vi "Robot Main.vi"() -> ()   [LabVIEW 2011]
doc: "This VI imlements the framework and scheduler for your robotics program. It should not be necessary to modify the framework. You are expected to add your code to the VIs called from Robot Main, the ones located in the Team Code within the project."
uses:
  <vilib>/Rock Robotics/WPI/Camera/WPI_CameraImageSize.ctl
  Robot Global Data.vi
panel:
  in  "Image Size":T1=enum."320x240"
  in  "Enable Vision":bool=TRUE
  in  "Finish":bool
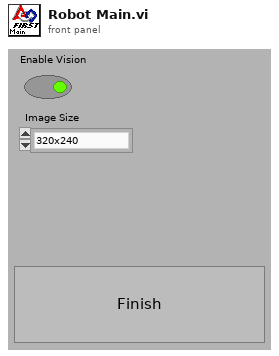
[diagram p1: front panel]
types:
  T1 = typedef "WPI_CameraImageSize.ctl" = enum16{"640x480", "320x240", "160x120"}
  T2 = typedef "WPI_DriverStationMatch Info.ctl" = cluster{"Autonomous Elapsed Seconds":dbl, "TeleOp Elapsed Seconds":dbl, "Disabled Elapsed Seconds":dbl, "Visited Autonomous":bool, "Visited TeleOp":bool, "Visited Disabled":bool, "Autonomous Settings":cluster{"Autonomous Style":enum16{"Iterative", "Independent"}, "VI Refnum":refnum<vi>}}
  T3 = typedef "WPI_DriverStationDerivedRobotMode.ctl" = enum16{"Init", "Execute", "Stop"}
  T4 = typedef "WPI_DriverStationRobotMode.ctl" = enum16{"Autonomous Disabled", "Autonomous Enabled", "Teleop Disabled", "Teleop Enabled", "Timeout", "Finish"}
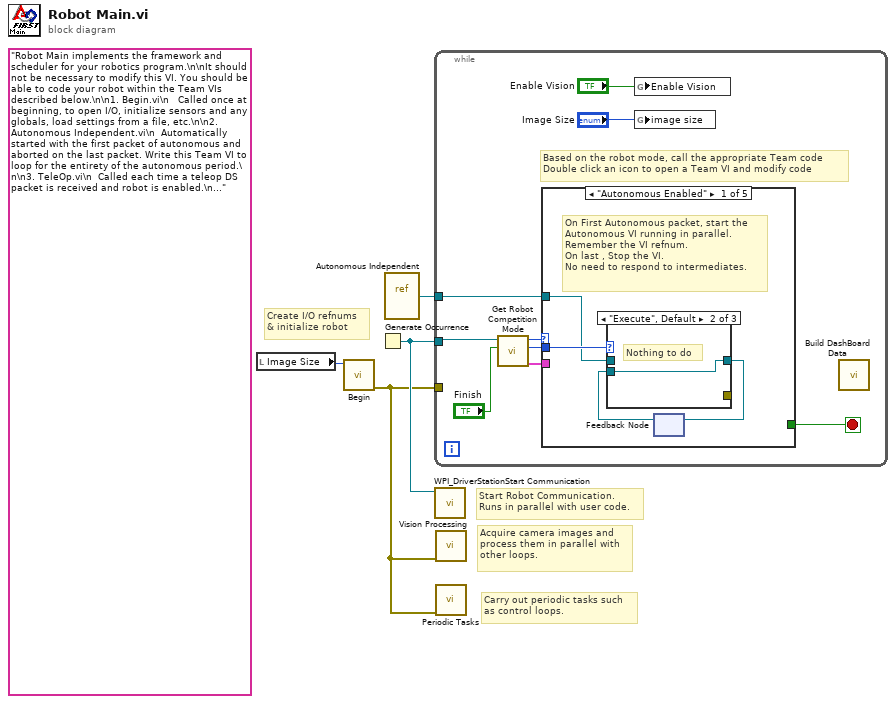
[diagram p0: block diagram]
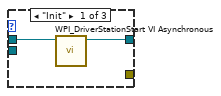
[diagram p2: hidden frame]
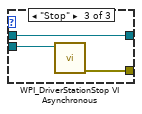
[diagram p3: hidden frame]
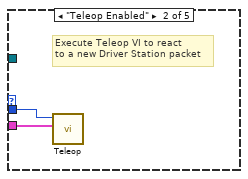
[diagram p4: hidden frame]
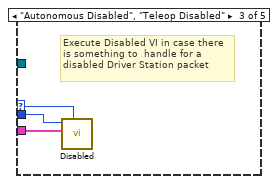
[diagram p5: hidden frame]
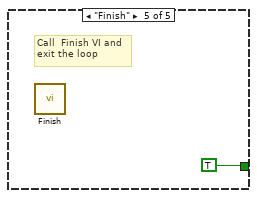
[diagram p7: hidden frame]
diagram:
  (unwired) "Robot Main implements the framework and scheduler for your robotics program.\n\nIt should not be necessary to modify this VI. You should be able to code your robot within the Team VIs described below.\n\n1. Begin.vi\n   Called once at beginning, to open I/O, initialize sensors and any globals, load settings from a file, etc.\n\n2. Autonomous Independent.vi\n  Automatically started with the first packet of autonomous and aborted on the last packet. Write this Team VI to loop for the entirety of the autonomous period.\n\n3. TeleOp.vi\n  Called each time a teleop DS packet is received and robot is enabled.\n\n4. Disabled.vi\n  Called each time a packet is received and the robot is disabled.\n\n5. Vision.vi\n  A parallel loop that acquires and processes camera images.\n\n6. PeriodicTasks.vi\n  Parallel loops running at user-defined rates.\n\n7. Finish.vi\n  Called before exiting, so you can save data, clean up I/O, etc.\n\n8. Build DashBoard Data.vi\n  Called for each driver station packet including timeouts. It is used to send select I/O values back to the Dashboard."
  # "Carry out periodic tasks such\nas control loops."
  # "Acquire camera images and\nprocess them in parallel with\nother loops."
  # "Create I/O refnums\n& initialize robot"
  # "Start Robot Communication.\nRuns in parallel with user code."
  n1 = local read "Image Size"() -> (w3:T1)
  n2 = call "Begin.vi"("Image Size"=w3) -> ("error out"=w1:errorcluster)  [unwired: 10 out]
  n3 = Generate Occurrence() -> (w4:refnum<k4>)
  n4 = vi-ref "Autonomous Independent.vi"() -> (w2:refnum<vi>)
  n5 = while {
    tunnel: w4 -> [w11]
    tunnel: w1 -> [_]
    tunnel: w2 -> [w6]
    stop <- w8 stop-if-true
    # "Based on the robot mode, call the appropriate Team code\nDouble click an icon to open a Team VI and modify code"
    n6 = call "Get Robot Competition Mode.vi"("Finish"="Finish", "DS Occurrence"=w11) -> ("Match Info out"=w9:T2, "Call Context"=w13:T3, "Robot Mode"=w12:T4)  [unwired: 7 out]
    n7 = case shown="\"Autonomous Enabled\"" w12 {
      selector: w12 -> [_ _ w26 _ _]
      tunnel: w13 -> [w17 w25 w28 _ _]
      tunnel: w9 -> [_ w24 w27 _ _]
      tunnel: [_ _ _ _ TRUE] -> w8
      tunnel: w6 -> [w16 _ _ _ _]
      frame "Autonomous Enabled" {
        # "On First Autonomous packet, start the\nAutonomous VI running in parallel.\nRemember the VI refnum.\nOn last , Stop the VI.\nNo need to respond to intermediates."
        n8 = feedback #1() -> (w14:refnum<vi>)  [unwired: 1 out]
        n9 = case shown="\"Execute\", Default" w17 {
          tunnel: w16 -> [w19 _ w22]
          tunnel: [w18 w20 w22] -> w15
          tunnel: w14 -> [_ w20 w23]
          tunnel: [_ _ w21] -> _
          frame "Init" {
            n10 = call <vilib>:"WPI_DriverStationStart VI Asynchronous.vi"("VI"=w19) -> ("VI out"=w18:refnum<vi>)  [unwired: 10 out]
          }
          frame "Execute", Default {
            # "Nothing to do"
          }
          frame "Stop" {
            n11 = call <vilib>:"WPI_DriverStationStop VI Asynchronous.vi"("VI Refnum"=w23) -> ("error out"=w21:errorcluster)  [unwired: 10 out]
          }
        }
        n12 = feedback-in #1(w15) -> ()
      }
      frame "Teleop Enabled" {
        # "Execute Teleop VI to react\nto a new Driver Station packet"
        n13 = call "Teleop.vi"("Match Info"=w24, "Call Context"=w25) -> ()  [unwired: 1 in, 9 out]
      }
      frame "Autonomous Disabled", "Teleop Disabled" {
        # "Execute Disabled VI in case there\nis something to  handle for a\ndisabled Driver Station packet"
        n14 = call "Disabled.vi"("Robot Mode"=w26, "Match Info"=w27, "Call Context"=w28) -> ()  [unwired: 1 in, 8 out]
      }
      frame "Timeout" {
        # "Driver Station packet didn't arrive.\nPossibly useful for diagnostics"
      }
      frame "Finish" {
        # "Call  Finish VI and\nexit the loop"
        n15 = call "Finish.vi"() -> ()  [unwired: 1 in, 7 out]
      }
    }
    n16 = global write "Robot Global Data.vi" "Enable Vision"("Enable Vision") -> ()
    n17 = global write "Robot Global Data.vi" "image size"("Image Size") -> ()
    n18 = call "Build DashBoard Data.vi"() -> ()  [unwired: 1 in, 11 out]
  }
  n19 = call <vilib>:"WPI_DriverStationStart Communication.vi"("occurrence"=w4) -> ()  [unwired: 11 out]
  n20 = call "Vision Processing.vi"("error in (no error)"=w1) -> ()  [unwired: 3 in, 4 out]
  n21 = call "Periodic Tasks.vi"("error in (no error)"=w1) -> ()  [unwired: 1 in, 10 out]
